vi "StartCountdown.vi"(1 "TimeoutName":string, 2 "TimeoutInterface":refnum<class "Timeout.lvclass">, 3 "TimeoutTime(s)":dbl, 5 "error in (no error)":errorcluster) -> (15 "TimeoutID":u32, 19 "error out":errorcluster)   [LabVIEW 2020, in "Timer.lvlib"]
uses:
  Timer.lvlib
  Timeout_interface/Timeout.lvclass
  TimeoutTask.vi
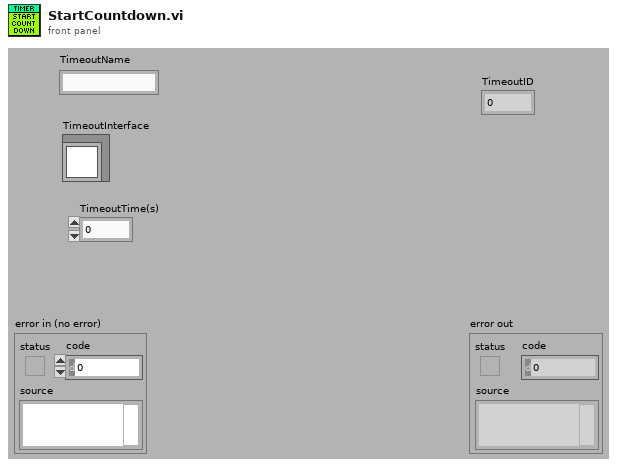
[diagram p1: front panel]
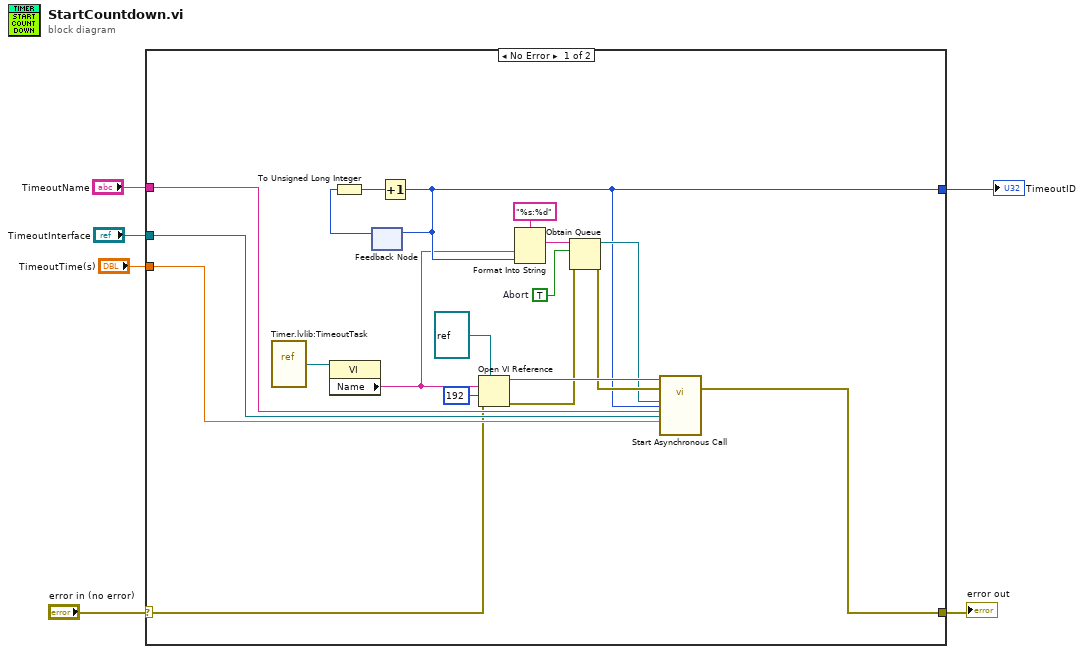
[diagram p0: block diagram]
diagram:
  n1 = case shown="No Error" "error in (no error)" {
    selector: "error in (no error)" -> [w8 w26]
    tunnel: [w9 w26] -> w5
    tunnel: [w13 _] -> w4
    tunnel: "TimeoutName" -> [w12 _]
    tunnel: "TimeoutInterface" -> [w11 _]
    tunnel: "TimeoutTime(s)" -> [w10 _]
    frame No Error {
      w21 = TRUE  # Abort
      n2 = vi-ref "Timer.lvlib:TimeoutTask.vi"() -> (w20:refnum<vi>)
      n3 = property class="VI"(reference=w20) -> ("Name"=w7:string)  [unwired: 1 in, 2 out]
      n4 = feedback #1() -> (w25:u32)  [unwired: 1 in]
      n5 = To Unsigned Long Integer(number=w25) -> (unsigned 32bit integer=w24:u32)
      n6 = Increment(x=w24) -> (x+1=w13:u32)
      n7 = feedback-in #1(w13) -> ()
      n8 = Open VI Reference(type specifier VI Refnum (for type only)=refnum<vi> refnum, vi path=w7, options=192, error in (no error)=w8) -> (vi reference=w17:refnum<vi>, error out=w16:errorcluster)  [unwired: 2 in]
      n9 = Format Into String(format string="%s:%d", w7, w13) -> (resulting string=w22:string)  [unwired: 2 in, 1 out]
      n10 = Obtain Queue(name (unnamed)=w22, element data type=w21, error in (no error)=w16) -> (queue out=w14:refnum<queue>, error out=w15:errorcluster)  [unwired: 2 in, 1 out]
      n11 = call-by-ref "Start Asynchronous Call"(reference=w17, error in=w15, "AbortQueue"=w14, "TimeoutID"=w13, "TimeoutName"=w12, "TimeoutInterface"=w11, "TimeoutTime(s)"=w10) -> (error out=w9:errorcluster)  [unwired: 14 in, 2 out]
    }
    frame Error {
    }
  }
  "error out" <- w5
  "TimeoutID" <- w4
